vi "BallShear_BallShear.vi"(8 "Check":bool, 11 "Selected Balls":dbl[][](array[numeric])) -> (0 "Ready":bool, 3 "Status":string)   [LabVIEW 2013]
panel:
  out "Selected Balls 2":dbl[][](array[numeric])
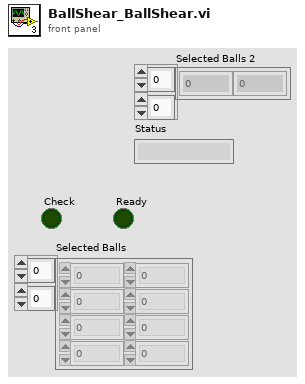
[diagram p1: front panel]
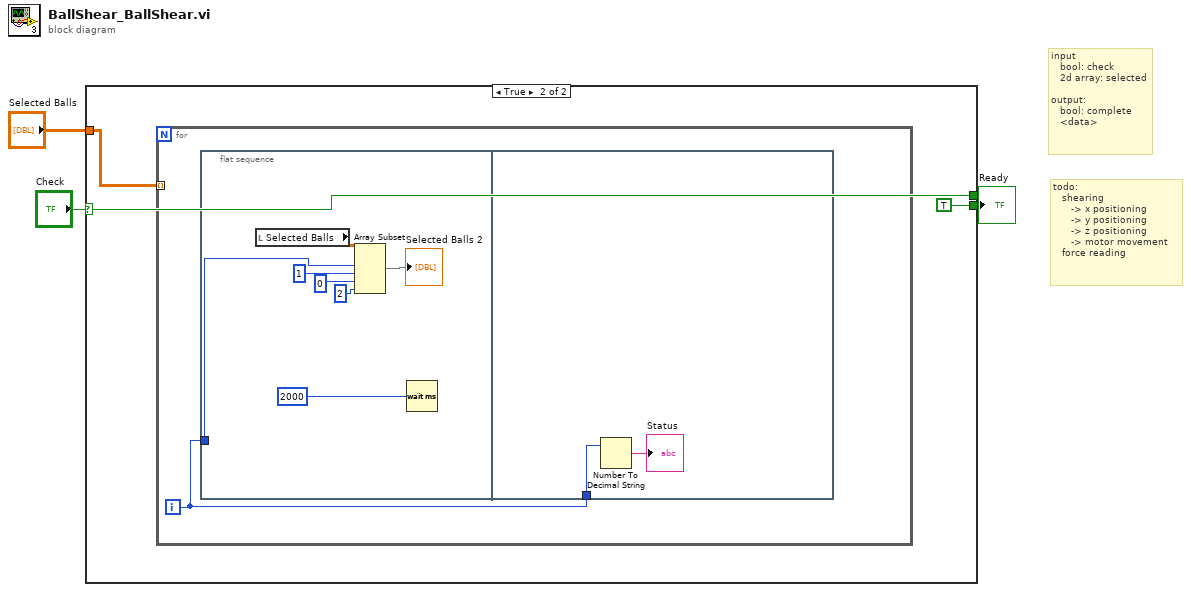
[diagram p0: block diagram]
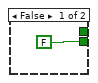
[diagram p2: hidden frame]
diagram:
  # "todo:\n   shearing\n      -> x positioning\n      -> y positioning\n      -> z positioning\n      -> motor movement\n   force reading"
  # "input\n   bool: check\n   2d array: selected\n\noutput:\n   bool: complete\n   <data>"
  n1 = case shown="True" "Check" {
    tunnel: "Check" -> [_ _]
    tunnel: [FALSE ("Power") TRUE ("Power")] -> w2
    tunnel: "Selected Balls" -> [_ w5]
    frame False {
    }
    frame True {
      n2 = for {
        tunnel: w5 -> [_] mode=indexing
        i -> [w7]
        n3 = flat-sequence {
          tunnel: w7 -> [w9]
          tunnel: w7 -> [w16]
          frame #0 {
            n4 = local read "Selected Balls"() -> (w10:dbl[][])
            n5 = Array Subset(array=w10, index (row)=w9, length (row)=1 ("length"), index (col)=0 ("index"), length (col)=2 ("length")) -> (→"Selected Balls 2":dbl[][])
            n6 = Wait (ms)(milliseconds to wait=u32 2000) -> ()  [unwired: 1 out]
          }
          frame #1 {
            n7 = Number To Decimal String(number=w16) -> (decimal integer string=→"Status":string)  [unwired: 1 in]
          }
        }
      }
    }
  }
  "Ready" <- w2
